vi "PhotonPipelineResult_CreateFromPacket.vi"(11 "RawData":u8[](array[numeric])) -> (3 "PhotonPipelineResult":T1 {"Targets"."Pose"."ROTATION"."SIN" format="%13.4f"; "Targets"."Pose"."ROTATION"."COS" format="%13.4f"; "Targets"."Pose"."ROTATION"."VALUE" format="%13.4f"; "Targets"."Pose"."TRANSLATION"."Y" format="%14.3f"; "Targets"."Pose"."TRANSLATION"."X" format="%14.3f"})   [LabVIEW 2019, in "PhotonVisionLib.lvlib"]
doc: "Internal function to parse the data returned by PhotonCamera_GetLatestResult.\n\nInputs:\n - RawData -- Byte array containing the data to parse.\n\nOutputs:\n - PipelineResult -- Parsed PipelineResult cluster."
uses:
  PhotonVisionLib.lvlib
  TypeDef/PhotonPipelineResultType.ctl
  TypeDef/PhotonTrackedTargetType.ctl
  TypeDef/TargetCornerType.ctl
  <vilib>/Rock Robotics/WPI/ThirdParty/JAS_Junk/TrajLib/POSE2D.ctl
  <vilib>/Rock Robotics/WPI/ThirdParty/JAS_Junk/TrajLib/TRANSLATION2D.ctl
  <vilib>/Rock Robotics/WPI/ThirdParty/JAS_Junk/TrajLib/ROTATION2D.ctl
  <vilib>/Rock Robotics/WPI/ThirdParty/JAS_Junk/TrajLib/Trajectory_Library.lvlib
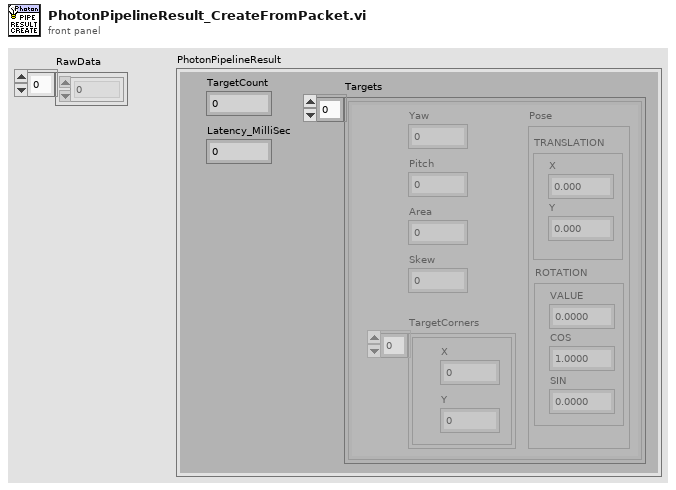
[diagram p1: front panel]
types:
  T1 = typedef "PhotonVisionLib.lvlib/PhotonPipelineResultType.ctl" = cluster{"TargetCount":i32, "Latency_MilliSec":dbl, "Targets":T2[]}
  T2 = typedef "PhotonVisionLib.lvlib/PhotonTrackedTargetType.ctl" = cluster{"Yaw":dbl, "Pitch":dbl, "Area":dbl, "Skew":dbl, "TargetCorners":T3[], "Pose":T4}
  T3 = typedef "PhotonVisionLib.lvlib/TargetCornerType.ctl" = cluster{"X":dbl, "Y":dbl}
  T4 = typedef "Trajectory_Library.lvlib/POSE2D.ctl" = cluster{"TRANSLATION":T5, "ROTATION":T6}
  T5 = typedef "Trajectory_Library.lvlib/TRANSLATION2D.ctl" = cluster{"X":dbl, "Y":dbl}
  T6 = typedef "Trajectory_Library.lvlib/ROTATION2D.ctl" = cluster{"VALUE":dbl, "COS":dbl, "SIN":dbl}
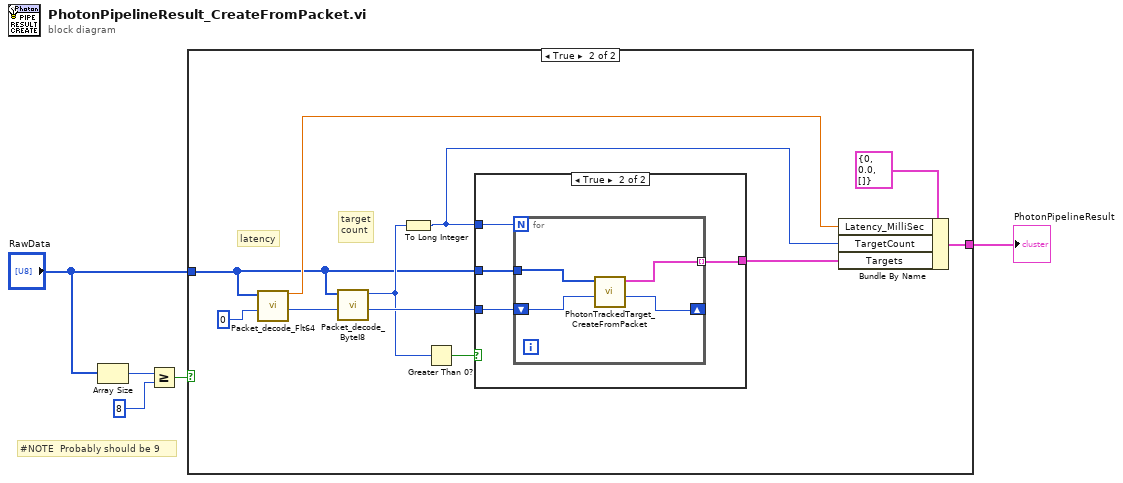
[diagram p0: block diagram]
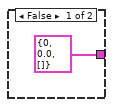
[diagram p2: hidden frame]
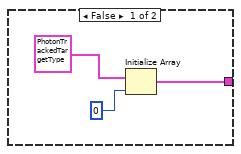
[diagram p3: hidden frame]
diagram:
  # "#NOTE  Probably should be 9"
  n1 = Array Size(array="RawData") -> (size(s)=w3:i32)
  n2 = Greater Or Equal?(x=w3, y=8) -> (x >= y?=w4:bool)
  n3 = case shown="True" w4 {
    tunnel: [T1 {"TargetCount"=0, "Latency_MilliSec"=0.0, "Targets"=[]} ("PhotonPipelineResult") w12] -> w5
    tunnel: "RawData" -> [_ w7]
    frame False {
    }
    frame True {
      # "target\ncount"
      # "latency"
      n4 = call "Packet_decode_Flt64.vi"("StartByte"=0, "RawData"=w7) -> ("NextByte"=w16:i32, "Flt64_Value"=w11:dbl)  [unwired: 8 in]
      n5 = call "Packet_decode_ByteI8.vi"("StartByte"=w16, "RawData"=w7) -> ("NextByte"=w14:i32, "Int8_Value"=w10:i8)  [unwired: 8 in]
      n6 = To Long Integer(number=w10) -> (32bit integer=w9:i32)
      n7 = Greater Than 0?(x=w10) -> (x > 0?=w15:bool)
      n8 = case shown="True" w15 {
        tunnel: w14 -> [_ w24]
        tunnel: w7 -> [_ w23]
        tunnel: w9 -> [_ w22]
        tunnel: [w18 w21] -> w8
        frame False {
          n9 = Initialize Array(T2 {"Yaw"=0.0, "Pitch"=0.0, "Area"=0.0, "Skew"=0.0, "TargetCorners"=[], "Pose"={"TRANSLATION"={"X"=0.0, "Y"=0.0}, "ROTATION"={"VALUE"=0.0, "COS"=1.0, "SIN"=0.0}}} ("PhotonTrackedTarget"), 0 ("dimension size")) -> (w18:T2[])
        }
        frame True {
          n10 = for {
            N: w22 -> [_]
            shift-right: [w25] -> _
            shift-left: w24 -> [w27]
            tunnel: w23 -> [w28]
            tunnel: [w26] -> w21 mode=indexing
            n11 = call "PhotonTrackedTarget_CreateFromPacket.vi"("StartByte"=w27, "RawData"=w28) -> ("NextByte"=w25:i32, "TrackedTarget"=w26:T2)  [unwired: 8 in]
          }
        }
      }
      n12 = Bundle By Name(cluster=T1 {"TargetCount"=0, "Latency_MilliSec"=0.0, "Targets"=[]} ("PhotonPipelineResult"), "Latency_MilliSec"=w11, "TargetCount"=w9, "Targets"=w8) -> (w12:T1)
    }
  }
  "PhotonPipelineResult" <- w5
